vi "imgrotate.vi"(10 "image data in":T1, 11 "transformation":T2(ring)) -> (3 "image data out":T1)   [LabVIEW 2023]
uses:
  <vilib>/picture/picture.llb/imagedata.ctl
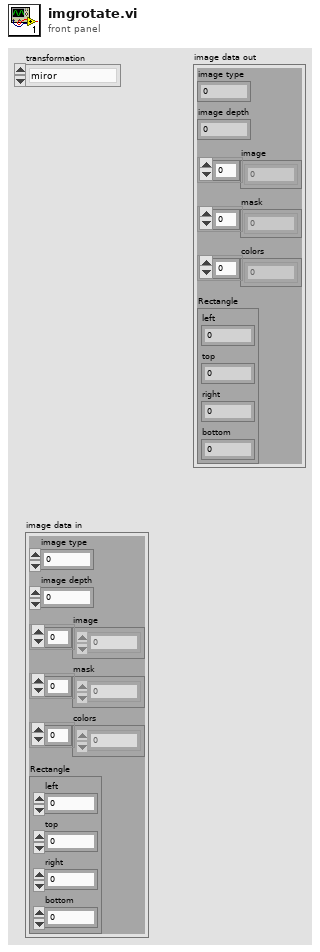
[diagram p1: front panel]
types:
  T1 = typedef "imagedata.ctl" = cluster{"image type":i32, "image depth":i32, "image":u8[], "mask":u8[], "colors":u32[], "Rectangle":cluster{"left":i16, "top":i16, "right":i16, "bottom":i16}}
  T2 = enum16{"miror", "rotate 0°", "rotate 90°", "rotate 180°", "rotate 270°"}
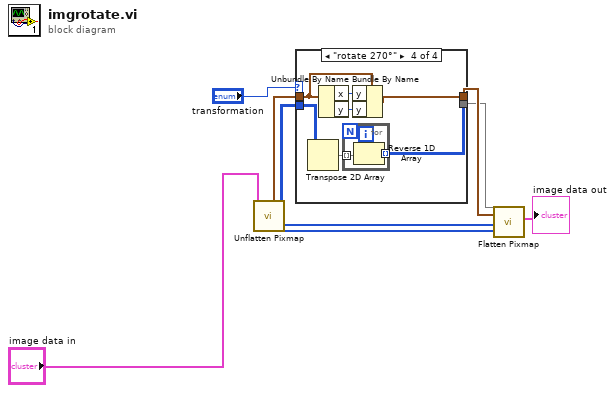
[diagram p0: block diagram]
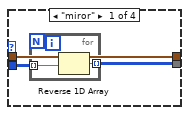
[diagram p2: hidden frame]
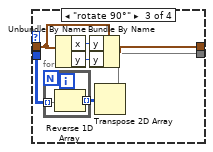
[diagram p4: hidden frame]
diagram:
  n1 = call <vilib>:"Unflatten Pixmap.vi"("image data"="image data in") -> ("24-bit pixmap"=w5:u32[][], "colors"=w2:u32[], "top left"=w8:cluster{"x":i16, "y":i16}, "mask"=w3:u8[])  [unwired: 4 in, 3 out]
  n2 = case shown="\"rotate 270°\"" "transformation" {
    tunnel: w5 -> [w12 w15 w19 w26]
    tunnel: [w11 w15 w17 w28] -> w6
    tunnel: w8 -> [w10 w16 w23 w32]
    tunnel: [w10 w16 w20 w29] -> w9
    frame "miror" {
      n3 = for {
        tunnel: w12 -> [w14] mode=indexing
        tunnel: [w13] -> w11 mode=indexing
        n4 = Reverse 1D Array(array=w14) -> (reversed array=w13:u32[])
      }
    }
    frame "rotate 0°", Default {
    }
    frame "rotate 90°" {
      n5 = for {
        tunnel: w19 -> [w25] mode=indexing
        tunnel: [w24] -> w18 mode=indexing
        n6 = Reverse 1D Array(array=w25) -> (reversed array=w24:u32[])
      }
      n7 = Unbundle By Name(w23) -> ("x"=w22:i16, "y"=w21:i16)
      n8 = Bundle By Name(cluster=w23, "y"=w22, "y"=w21) -> (w20:cluster{"x":i16, "y":i16})
      n9 = Transpose 2D Array(2D array=w18) -> (transposed array=w17:u32[][])
    }
    frame "rotate 270°" {
      n10 = Transpose 2D Array(2D array=w26) -> (transposed array=w27:u32[][])
      n11 = Unbundle By Name(w32) -> ("x"=w31:i16, "y"=w30:i16)
      n12 = for {
        tunnel: w27 -> [w34] mode=indexing
        tunnel: [w33] -> w28 mode=indexing
        n13 = Reverse 1D Array(array=w34) -> (reversed array=w33:u32[])
      }
      n14 = Bundle By Name(cluster=w32, "y"=w31, "y"=w30) -> (w29:cluster{"x":i16, "y":i16})
    }
  }
  n15 = call <vilib>:"Flatten Pixmap.vi"("mask"=w3, "colors"=w2, "top left"=w9, "24-bit pixmap"=w6) -> ("image data"=→"image data out":T1)  [unwired: 7 in]
